vi "WaveformArrayTo2DArray.vi"(11 "Waveform Array":waveform(dbl)[](array[waveform])) -> (3 "2-D Array":dbl[][](array[numeric]))   [LabVIEW 2016]
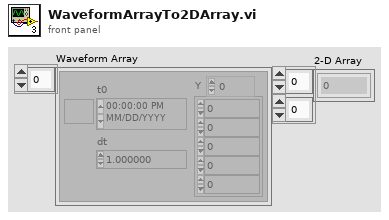
[diagram p1: front panel]
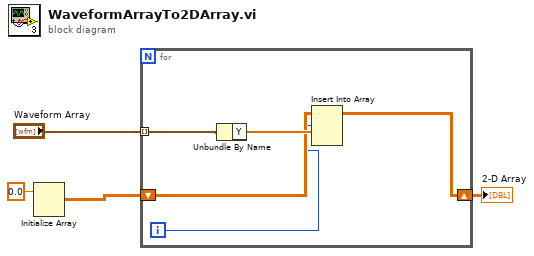
[diagram p0: block diagram]
diagram:
  n1 = Initialize Array(0.0 ("element")) -> (w2:dbl[][])  [unwired: 2 in]
  n2 = for {
    tunnel: "Waveform Array" -> [w9] mode=indexing
    shift-right: [w6] -> w1
    shift-left: w2 -> [w7]
    i -> [w5]
    n3 = Unbundle By Name(w9) -> ("Y"=w8:dbl[])
    n4 = Insert Into Array(array=w7, index (row)=w5, new element=w8) -> (w6:dbl[][])  [unwired: 1 in]
  }
  "2-D Array" <- w1
